vi "XY Persistent Data to Variant.vi"(8 "error in (no error)":errorcluster, 11 "Persistent Data":T1={"Label"="", "Graph Props"={"Plots"=[], "Legend:Number of Rows"=0, "Scale Properties"={"X.Auto"=FALSE, "X.Min"=0.0, "X.Max"=0.0, "X.IgnoreTS"=FALSE, "X.Precision"=0, "X.Label:"="", "X.LabelVis"=FALSE, "X.DefLabel"=FALSE, "Y.Auto"=FALSE, "Y.Min"=0.0, "Y.Max"=0.0, "Y.Format"=0, "Y.Precision:"=0, "Y.Label:"="", "Y.LabelVis"=FALSE, "Y.DefLabel"=FALSE, "X.Format"=0}, "Legend:Visible"=TRUE, "BgColor"=0, "Last Plot Width"=0, "Resize"=FALSE}, "UDP Data"={"Decimation"=0, "UDP Buffer Size"=0, "History Length"=0.0, "Update Rate"=enum."15 Hz", "Channel Paths"=[], "Channel Names"=[]}} {"Graph Props"."Scale Properties"."X.Format" items=["Decimal", "Scientific", "Engineering", "Binary", "Octal", "Hexadecimal", "Relative Time", "Time and Date", "SI", "Automatic"]; "Graph Props"."Scale Properties"."Y.Precision:" items=["0", "1", "2", "3", "4", "5", "6", "7"]; "Graph Props"."Scale Properties"."Y.Format" items=["Decimal", "Scientific", "Engineering", "Binary", "Octal", "Hexadecimal", "Relative Time", "Time and Date", "SI", "Automatic"]; "Graph Props"."Scale Properties"."X.Precision" items=["0", "1", "2", "3", "4", "5", "6", "7"]}) -> (0 "error out":errorcluster, 3 "Variant":variant)   [LabVIEW 2020, in "Workspace MultiY Graph.lvlib"]
uses:
  Workspace MultiY Graph.lvlib
  XY Persistent Data.ctl
  XY Graph Properties.ctl
  XY Plot Properties.ctl
  XY Scale Properties.ctl
  XY Scale Precision.ctl
  XY Scale Format.ctl
  UDP Data.ctl
  Update Rate.ctl
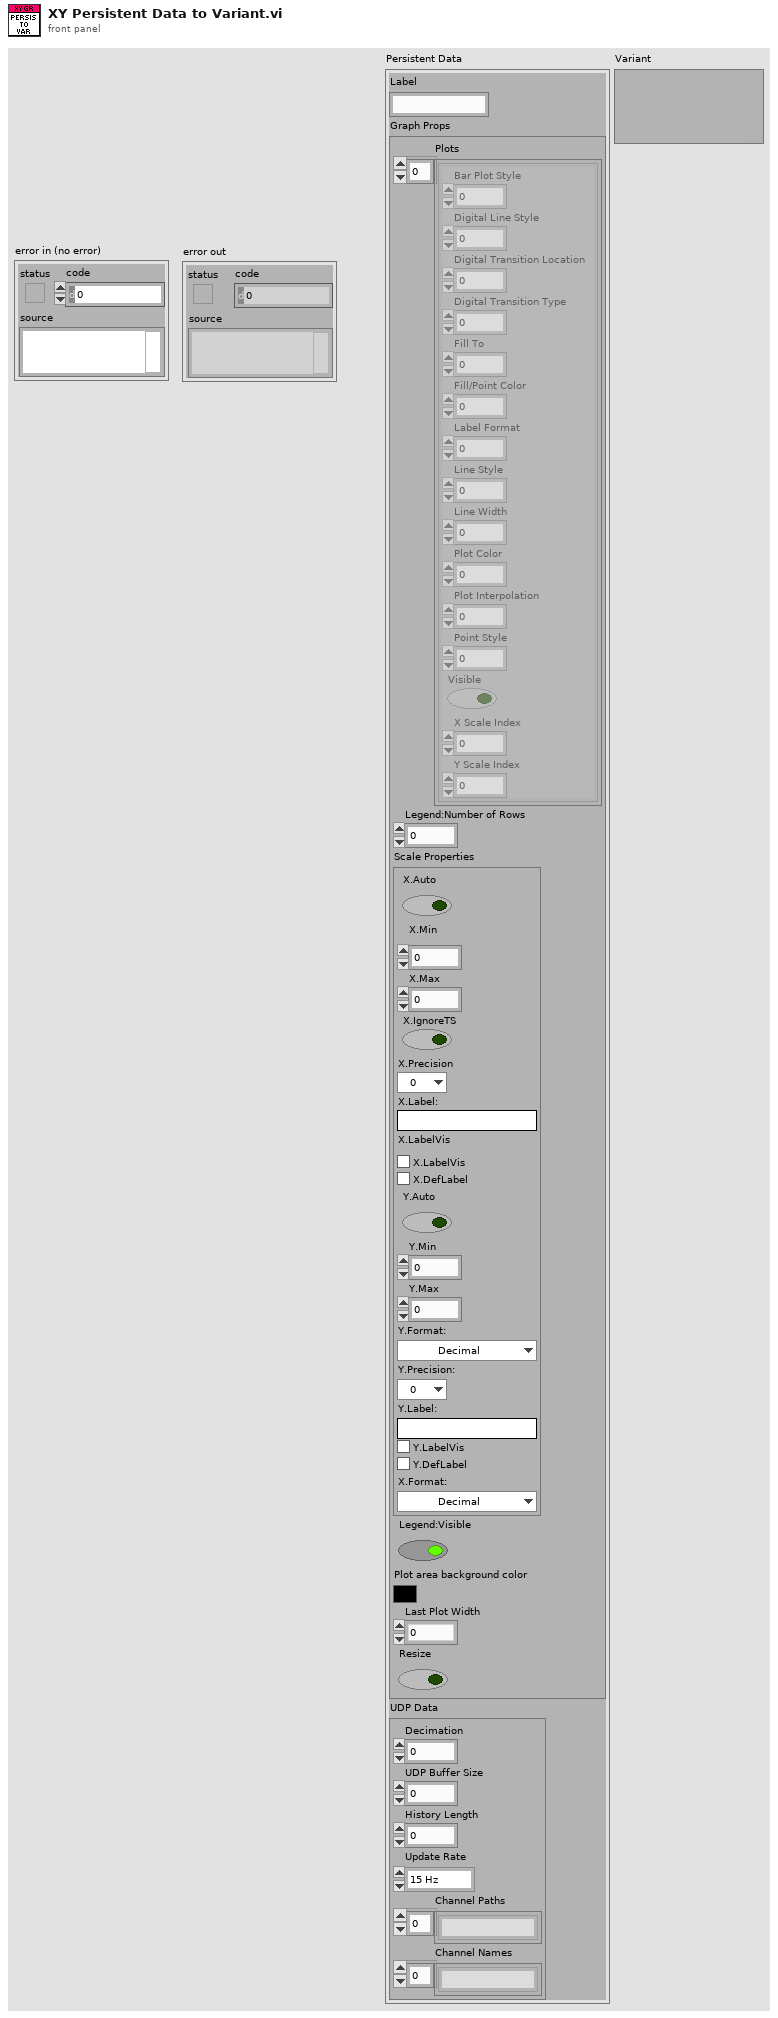
[diagram p1: front panel]
types:
  T1 = typedef "Workspace MultiY Graph.lvlib/XY Persistent Data.ctl" = cluster{"Label":string, "Graph Props":T2, "UDP Data":T7}
  T2 = typedef "Workspace MultiY Graph.lvlib/XY Graph Properties.ctl" = cluster{"Plots":T3[], "Legend:Number of Rows":u32, "Scale Properties":T4, "Legend:Visible":bool, "BgColor":u32, "Last Plot Width":u32, "Resize":bool}
  T3 = typedef "Workspace MultiY Graph.lvlib/XY Plot Properties.ctl" = cluster{"Bar Plot Style":u8, "Digital Line Style":u8, "Digital Transition Location":u8, "Digital Transition Type":u8, "Fill To":i16, "Fill/Point Color":u32, "Label Format":u8, "Line Style":u8, "Line Width":u8, "Plot Color":u32, "Plot Interpolation":u8, "Point Style":u8, "Visible":bool, "X Scale Index":u32, "Y Scale Index":u32}
  T4 = typedef "Workspace MultiY Graph.lvlib/XY Scale Properties.ctl" = cluster{"X.Auto":bool, "X.Min":dbl, "X.Max":dbl, "X.IgnoreTS":bool, "X.Precision":T5, "X.Label:":string, "X.LabelVis":bool, "X.DefLabel":bool, "Y.Auto":bool, "Y.Min":dbl, "Y.Max":dbl, "Y.Format":T6, "Y.Precision:":T5, "Y.Label:":string, "Y.LabelVis":bool, "Y.DefLabel":bool, "X.Format":T6}
  T5 = typedef "Workspace MultiY Graph.lvlib/XY Scale Precision.ctl" = u8
  T6 = typedef "Workspace MultiY Graph.lvlib/XY Scale Format.ctl" = u8
  T7 = typedef "Workspace MultiY Graph.lvlib/UDP Data.ctl" = cluster{"Decimation":i32, "UDP Buffer Size":u32, "History Length":dbl, "Update Rate":T8, "Channel Paths":string[], "Channel Names":string[]}
  T8 = typedef "Workspace MultiY Graph.lvlib/Update Rate.ctl" = enum8{"15 Hz", "10 Hz", "5 Hz", "4 Hz", "3 Hz", "2 Hz", "1 Hz", "0.5 Hz"}
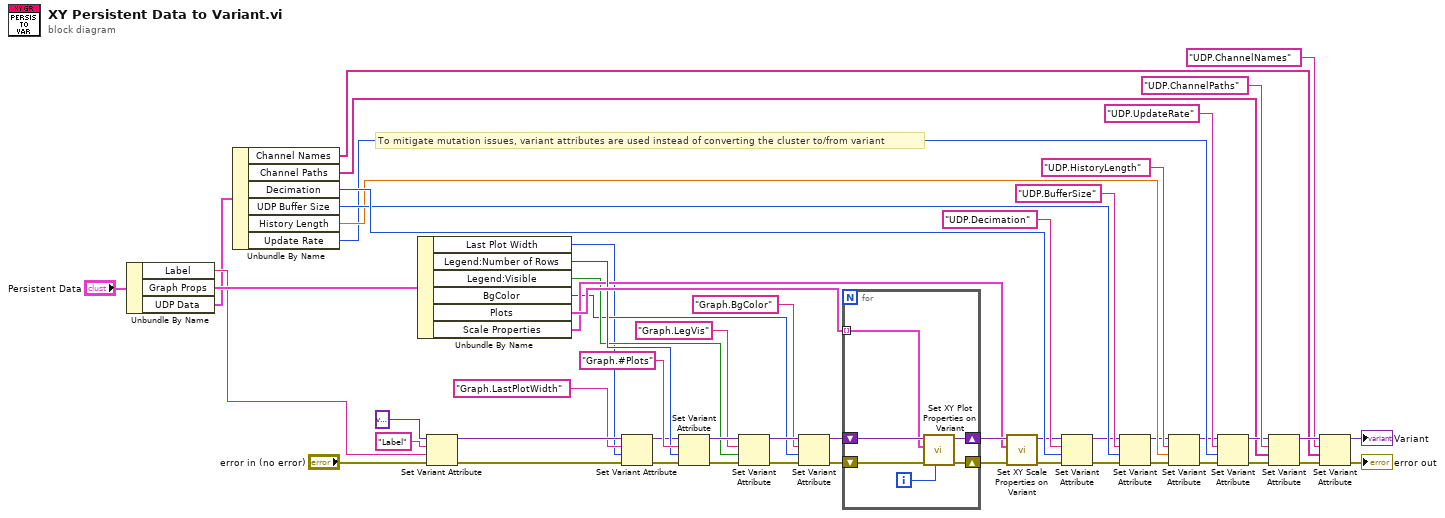
[diagram p0: block diagram]
diagram:
  # "To mitigate mutation issues, variant attributes are used instead of converting the cluster to/from variant"
  n1 = Unbundle By Name("Persistent Data") -> ("Label"=w50:string, "Graph Props"=w51:T2, "UDP Data"=w27:T7)
  n2 = Unbundle By Name(w27) -> ("Channel Names"=w3:string[], "Channel Paths"=w9:string[], "Decimation"=w25:i32, "UDP Buffer Size"=w23:u32, "History Length"=w21:dbl, "Update Rate"=w20:T8)
  n3 = Unbundle By Name(w51) -> ("Last Plot Width"=w28:u32, "Legend:Number of Rows"=w47:u32, "Legend:Visible"=w40:bool, "BgColor"=w34:u32, "Plots"=w49:T3[], "Scale Properties"=w44:T4)
  n4 = Set Variant Attribute(Variant=variant ("variant"), name="Label", value=w50, error in="error in (no error)") -> (Variant out=w30:variant, error out=w31:errorcluster)  [unwired: 1 out]
  n5 = Set Variant Attribute(Variant=w30, name="Graph.LastPlotWidth", value=w28, error in=w31) -> (Variant out=w32:variant, error out=w33:errorcluster)  [unwired: 1 out]
  n6 = Set Variant Attribute(Variant=w32, name="Graph.#Plots", value=w47, error in=w33) -> (Variant out=w42:variant, error out=w43:errorcluster)  [unwired: 1 out]
  n7 = Set Variant Attribute(Variant=w42, name="Graph.LegVis", value=w40, error in=w43) -> (Variant out=w36:variant, error out=w37:errorcluster)  [unwired: 1 out]
  n8 = Set Variant Attribute(Variant=w36, name="Graph.BgColor", value=w34, error in=w37) -> (Variant out=w38:variant, error out=w39:errorcluster)  [unwired: 1 out]
  n9 = for {
    shift-right: [w60] -> w45
    shift-left: w38 -> [w61]
    shift-right: [w59] -> w46
    shift-left: w39 -> [w58]
    tunnel: w49 -> [w57] mode=indexing
    i -> [w56]
    n10 = call "Set XY Plot Properties on Variant.vi"("Plot#"=w56, "error in (no error)"=w58, "Plot"=w57, "variant in"=w61) -> ("error out"=w59:errorcluster, "variant out"=w60:variant)  [unwired: 6 in]
  }
  n11 = call "Set XY Scale Properties on Variant.vi"("error in (no error)"=w46, "Scale Properties"=w44, "variant in"=w45) -> ("error out"=w1:errorcluster, "variant out"=w2:variant)  [unwired: 7 in]
  n12 = Set Variant Attribute(Variant=w2, name="UDP.Decimation", value=w25, error in=w1) -> (Variant out=w17:variant, error out=w16:errorcluster)  [unwired: 1 out]
  n13 = Set Variant Attribute(Variant=w17, name="UDP.BufferSize", value=w23, error in=w16) -> (Variant out=w15:variant, error out=w14:errorcluster)  [unwired: 1 out]
  n14 = Set Variant Attribute(Variant=w15, name="UDP.HistoryLength", value=w21, error in=w14) -> (Variant out=w13:variant, error out=w12:errorcluster)  [unwired: 1 out]
  n15 = Set Variant Attribute(Variant=w13, name="UDP.UpdateRate", value=w20, error in=w12) -> (Variant out=w11:variant, error out=w10:errorcluster)  [unwired: 1 out]
  n16 = Set Variant Attribute(Variant=w11, name="UDP.ChannelPaths", value=w9, error in=w10) -> (Variant out=w7:variant, error out=w8:errorcluster)  [unwired: 1 out]
  n17 = Set Variant Attribute(Variant=w7, name="UDP.ChannelNames", value=w3, error in=w8) -> (Variant out=→"Variant":variant, error out=→"error out":errorcluster)  [unwired: 1 out]
